vi "getSortedRow.vi"(10 "index (row)":i32, 11 "Array":dbl[][](array[numeric])) -> (3 "sorted array":dbl[](array[numeric]))   [LabVIEW 2017]
doc: "Replaces row at index with another row"
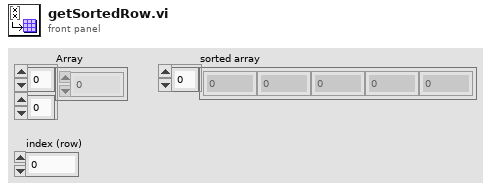
[diagram p1: front panel]
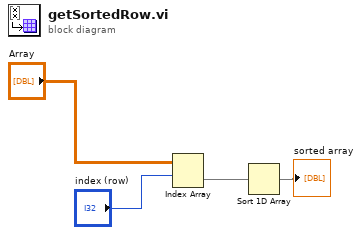
[diagram p0: block diagram]
diagram:
  n1 = Index Array(array="Array", index (row)="index (row)") -> (element=w3:dbl[])  [unwired: 1 in]
  n2 = Sort 1D Array(array=w3) -> (sorted array=→"sorted array":dbl[])
